vi "PI_GCS2_Sample_Application_Motion.vi"() -> ()   [LabVIEW 2020]
doc: "This VI demonstrates how to initialize a PI GCS2 system and how to query the help answer. \nThe diagram shows how to combine the driver VIs for these tasks. \n\nWarning: Before running this VI, modify the interface settings on the block diagram to reflect your configuration. The predefined settings provided with the VI probably do not match your system."
uses:
  Interface Settings.ctl
panel:
  out "All axes on target?":bool
  out "All axes referenced?":bool
  out "Axes available?":bool caption="Any axes available?"
  out "Axis on target?":bool[](array[boolean])
  out "Referenced?":bool[](array[boolean])
  out "Any axes moving?":bool
  in  "Target Position":dbl[](array[numeric]) format="%.6f"
  out "Current Position":dbl[](array[numeric]) format="%.6f"
  in  "stop":bool
  in  "error in":errorcluster
  out "Running":bool caption="Configuration_Setup.vi is running"
  out "error out":errorcluster
  out "Conn. Axis":string[](array[string])
  out "Identification":string
  # "This VI demonstrates how to initialize a PI GCS2 system and how to move your axes.\nThe diagram shows how to combine the driver VIs for these tasks. \n\nWarning: Before running this VI, modify the interface settings on the block diagram to reflect your configuration.\n                 The predefined settings provided with the VI probably do not match your system.\n\nCompatibility: This sample will not work with E-518 controllers."
  # "Set the number of target positions\naccording to your connected axes."
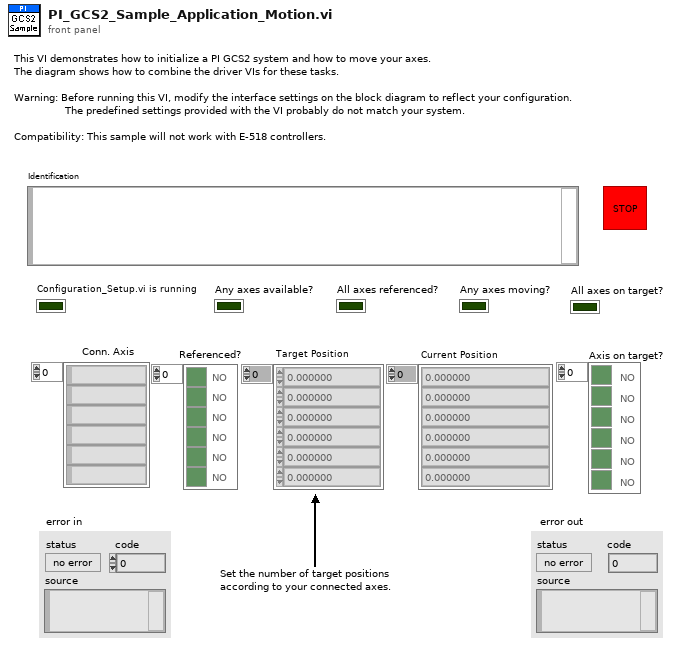
[diagram p1: front panel]
types:
  T1 = typedef "Interface Settings.ctl" = cluster{"Interface":u16, "Timeout":u32, "RS232 settings":cluster{"Portnumber":u8, "Baudrate":u16}, "TCP/IP settings":cluster{"Host address/name":string, "Port":i32, "Board":i32, "TCP/IP Search?":bool}, "USB settings":cluster{"S/N":string, "USB Search?":bool}, "DaisyChain settings":cluster{"Register DC":bool, "DaisyChain Search?":bool, "Device ID":i32}, "DLL for Device":u16}
  T2 = enum16{"Do not reference", "Reference switch", "Negative limit switch", "Positive limit switch"}[]
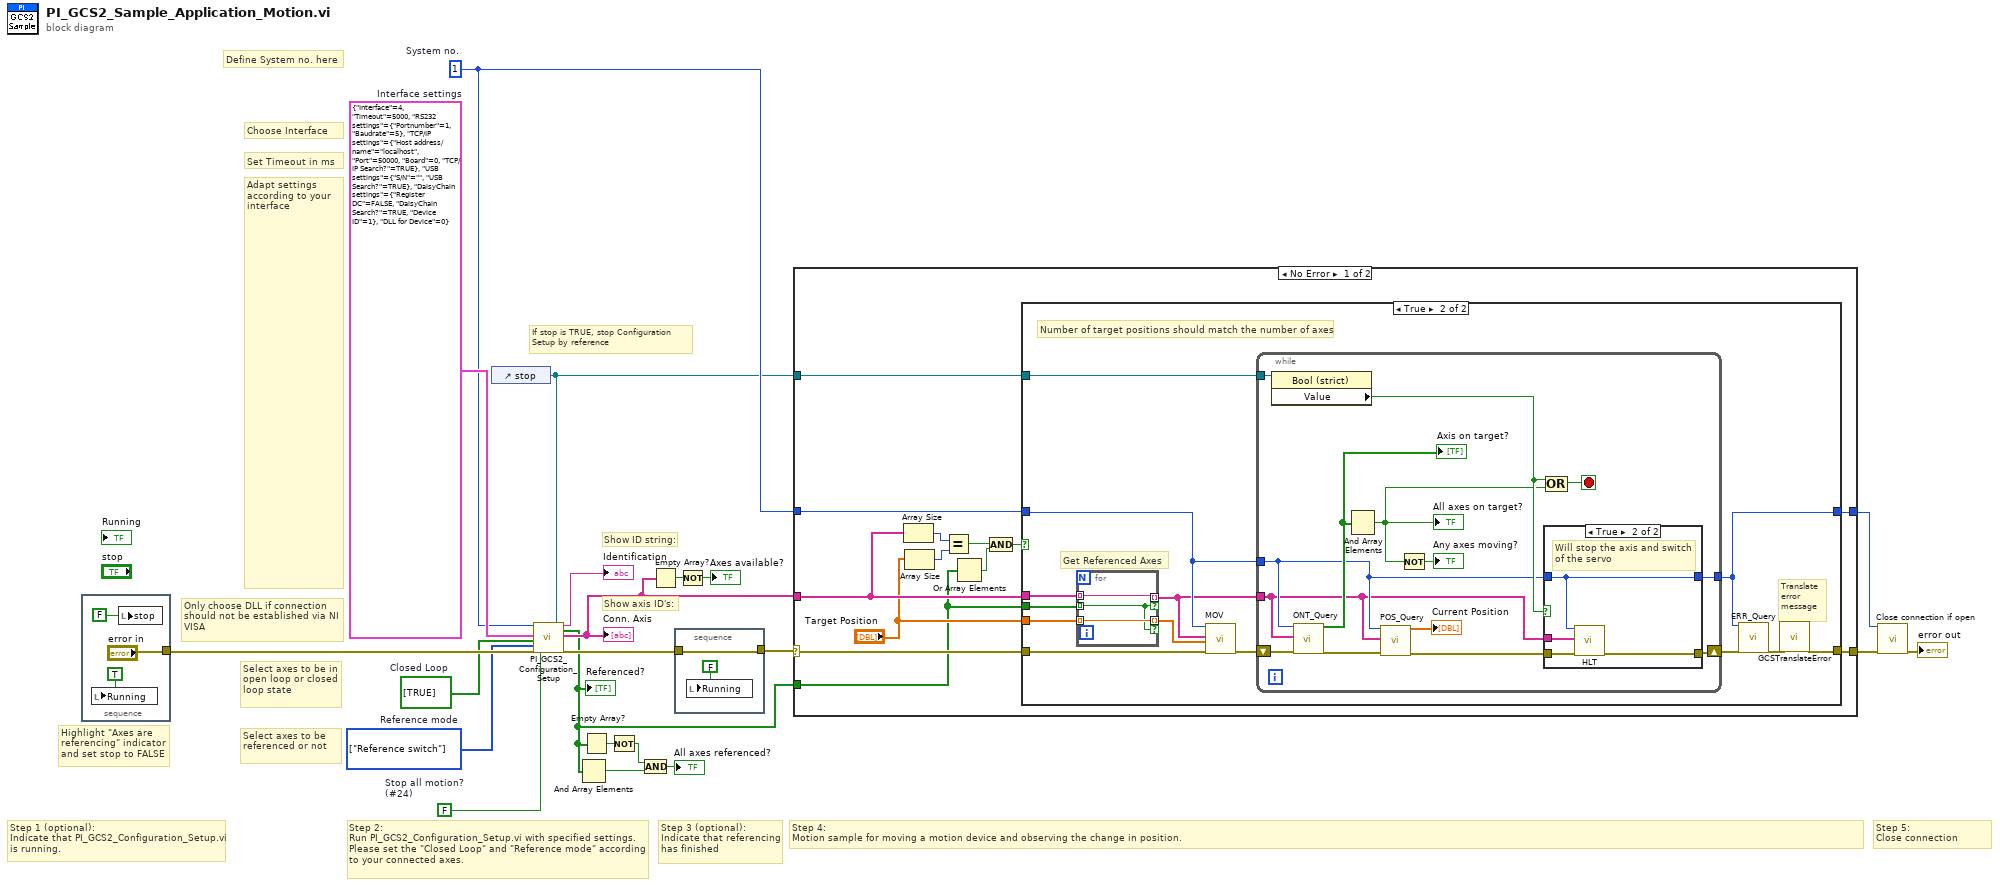
[diagram p0: block diagram]
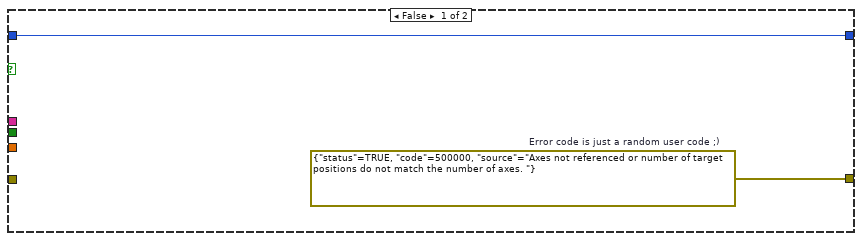
[diagram p2: hidden frame]
diagram:
  w14 = T1 {"Interface"=4, "Timeout"=5000, "RS232 settings"={"Portnumber"=1, "Baudrate"=5}, "TCP/IP settings"={"Host address/name"="localhost", "Port"=50000, "Board"=0, "TCP/IP Search?"=TRUE}, "USB settings"={"S/N"="", "USB Search?"=TRUE}, "DaisyChain settings"={"Register DC"=FALSE, "DaisyChain Search?"=TRUE, "Device ID"=1}, "DLL for Device"=0}  # Interface settings
  w15 = FALSE  # Stop all motion? (#24)
  w16 = T2 [enum."Reference switch"] items=["Do not reference", "Reference switch", "Negative limit switch", "Positive limit switch"]  # Reference mode
  w17 = bool[] [TRUE]  # Closed Loop
  w11 = 1  # System no.
  # "Step 5:\nClose connection"
  # "Define System no. here"
  # "Select axes to be referenced or not"
  # "Select axes to be in open loop or closed loop state"
  # "Adapt settings according to your interface"
  # "Set Timeout in ms"
  # "Choose Interface"
  # "Only choose DLL if connection should not be established via NI VISA"
  # "If stop is TRUE, stop Configuration\nSetup by reference"
  # "Step 4: \nMotion sample for moving a motion device and observing the change in position."
  # "Step 3 (optional): \nIndicate that referencing has finished"
  # "Step 2: \nRun PI_GCS2_Configuration_Setup.vi with specified settings.\nPlease set the \"Closed Loop\" and \"Reference mode\" according\nto your connected axes."
  # "Step 1 (optional): \nIndicate that PI_GCS2_Configuration_Setup.vi is running."
  # "Highlight \"Axes are\nreferencing\" indicator\nand set stop to FALSE"
  # "Show axis ID's:"
  # "Show ID string:"
  n1 = stacked-sequence {
    tunnel: ["error in"] -> w20
    frame #0 {
      n2 = local write "Running"(TRUE ("Running")) -> ()
      n3 = local write "stop"(FALSE ("stop")) -> ()
    }
  }
  n4 = control-ref of="stop"() -> (w10:refnum<vi>)
  n5 = call "PI_GCS2_Configuration_Setup.vi"("System no."=w11, "Interface settings"=w14, "Closed Loop"=w17, "Reference mode"=w16, "error in"=w20, "Stop all motion?"=w15, "Stop refnum"=w10) -> ("Identification"=→"Identification":string, "Referenced?"=w4:bool[], "Conn. Axis"=w6:string[], "error out"=w19:errorcluster)  [unwired: 1 in, 8 out]
  "Conn. Axis" <- w6
  "Referenced?" <- w4
  n6 = And Array Elements(Boolean array=w4) -> (logical AND=w1:bool)
  n7 = Empty Array?(array=w4) -> (empty?=w5:bool)
  n8 = Not(x=w5) -> (.not. x?=w2:bool)
  n9 = And(x=w2, y=w1) -> (x .and. y?=→"All axes referenced?":bool)
  n10 = Empty Array?(array=w6) -> (empty?=w8:bool)
  n11 = stacked-sequence {
    tunnel: w19 -> [w25]
    tunnel: [w25] -> w13
    frame #0 {
      n12 = local write "Running"(FALSE ("Running")) -> ()
    }
  }
  n13 = Not(x=w8) -> (.not. x?=→"Axes available?":bool)
  n14 = case shown="No Error" w13 {
    selector: w13 -> [w28 w79]
    tunnel: [w39 w79] -> w9
    tunnel: w11 -> [w37 w78]
    tunnel: [w38 w78] -> w12
    tunnel: w6 -> [w35 _]
    tunnel: w10 -> [w36 _]
    tunnel: w4 -> [w27 _]
    frame No Error {
      n15 = Array Size(array=w35) -> (size(s)=w33:i32)
      n16 = Array Size(array="Target Position") -> (size(s)=w32:i32)
      n17 = Equal?(x=w33, y=w32) -> (x = y?=w31:bool)
      n18 = Or Array Elements(Boolean array=w27) -> (logical OR=w29:bool)
      n19 = And(x=w31, y=w29) -> (x .and. y?=w30:bool)
      n20 = case shown="True" w30 {
        tunnel: [w40 w54] -> w39
        tunnel: w28 -> [_ w52]
        tunnel: [w41 w50] -> w38
        tunnel: w35 -> [_ w49]
        tunnel: w27 -> [_ w48]
        tunnel: w37 -> [w41 w47]
        tunnel: w36 -> [_ w45]
        tunnel: "Target Position" -> [_ w43]
        frame False {
          w40 = errorcluster {"status"=TRUE, "code"=500000, "source"="Axes not referenced or number of target positions do not match the number of axes. "}  # Error code is just a random user code ;)
        }
        frame True {
          # "Number of target positions should match the number of axes"
          # "Get Referenced Axes"
          # "Translate\nerror \nmessage"
          n21 = for {
            tunnel: w49 -> [w57] mode=indexing
            tunnel: w48 -> [w55] mode=indexing
            tunnel: [w57] -> w46 mode=indexing if=w55
            tunnel: [w56] -> w42 mode=indexing if=w55
            tunnel: w43 -> [w56] mode=indexing
          }
          n22 = call "MOV.vi"("System no."=w47, "Axes to move"=w46, "Position values"=w42, "error in"=w52) -> ("error out"=w44:errorcluster)  [unwired: 1 in, 14 out]
          n23 = while {
            shift-right: [w69] -> w51
            shift-left: w44 -> [w63]
            tunnel: w45 -> [w68]
            tunnel: w47 -> [w62]
            tunnel: w46 -> [w61]
            tunnel: [w64] -> w50
            stop <- w67 stop-if-true
            n24 = property class="Bool (strict)"(reference=w68) -> ("Value"=w66:bool)  [unwired: 1 in, 2 out]
            n25 = call "ONT_Query.vi"("System no."=w62, "Axes to query"=w61, "error in"=w63) -> ("Axis on target?"=w65:bool[], "error out"=w71:errorcluster)  [unwired: 2 in, 13 out]
            "Axis on target?" <- w65
            n26 = And Array Elements(Boolean array=w65) -> (logical AND=w58:bool)
            "All axes on target?" <- w58
            n27 = call "POS_Query.vi"("System no."=w62, "Axes to query"=w61, "error in"=w71) -> ("Position"=→"Current Position":dbl[], "error out"=w70:errorcluster)  [unwired: 2 in, 13 out]
            n28 = Not(x=w58) -> (.not. x?=→"Any axes moving?":bool)
            n29 = case shown="True" w66 {
              tunnel: w70 -> [w73 w76]
              tunnel: [w73 w75] -> w69
              tunnel: w62 -> [w72 w77]
              tunnel: [w72 w77] -> w64
              tunnel: w61 -> [_ w74]
              frame False {
              }
              frame True {
                # "Will stop the axis and switch of the servo"
                n30 = call "HLT.vi"("System no."=w77, "Affected axes"=w74, "error in"=w76) -> ("error out"=w75:errorcluster)  [unwired: 16 in]
              }
            }
            n31 = Compound Arithmetic op=OR(w66, w58) -> (w67:bool)
          }
          n32 = call "ERR_Query.vi"("System no."=w50, "error in"=w51) -> ("error out"=w53:errorcluster)  [unwired: 17 out]
          n33 = call "GCSTranslateError.vi"("error in"=w53) -> ("error out"=w54:errorcluster)  [unwired: 18 out]
        }
      }
    }
    frame Error {
      # "Error during initialization"
    }
  }
  n34 = call "Close connection if open.vi"("System no."=w12, "error in"=w9) -> ("error out"=→"error out":errorcluster)  [unwired: 1 in, 16 out]
